vi "Read Shared Library.vi"(8 "Error In":errorcluster, 11 "SFTP In":refnum<class "SFTP.lvclass">) -> (0 "Erorr Out":errorcluster, 2 "libssh2lv Shared Library":path, 3 "SFTP Out":refnum<class "SFTP.lvclass">)   [LabVIEW 2018, in "Toolkit.lvlib" / "SFTP.lvclass"]
uses:
  SFTP.lvclass
  SFTP.lvclass/SFTP.ctl
  Session/Session.lvclass/Session.ctl
  SSH/SSH.lvclass/SSH.ctl
  Session/Session.lvclass
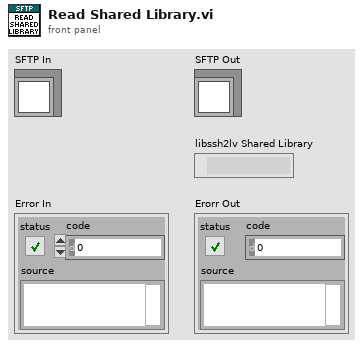
[diagram p1: front panel]
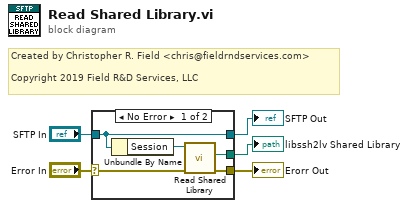
[diagram p0: block diagram]
diagram:
  # "Created by Christopher R. Field <chris@fieldrndservices.com>\n\nCopyright 2019 Field R&D Services, LLC"
  n1 = case shown="No Error" "Error In" {
    selector: "Error In" -> [w8 w11]
    tunnel: [w7 w11] -> w4
    tunnel: "SFTP In" -> [w10 w12]
    tunnel: [w10 w12] -> w2
    tunnel: [w6 _] -> w1
    frame No Error {
      n2 = Unbundle By Name(w10) -> ("Session"=w9:refnum<class "Session.lvclass">)
      n3 = call "Read Shared Library.vi"("Error In"=w8, "Session In"=w9) -> ("Erorr Out"=w7:errorcluster, "libssh2lv Shared Library"=w6:path)  [unwired: 7 in, 1 out]
    }
    frame Error {
    }
  }
  "Erorr Out" <- w4
  "SFTP Out" <- w2
  "libssh2lv Shared Library" <- w1
